vi "disk.vi"() -> ()   [LabVIEW 2016]
panel:
  out "free (bytes)":i64
  out "error out":errorcluster
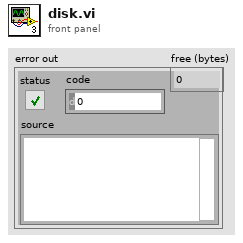
[diagram p1: front panel]
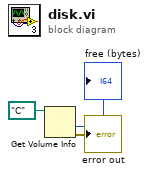
[diagram p0: block diagram]
diagram:
  n1 = Get Volume Info(11:path "C:/" ("path")) -> (0:→"error out":errorcluster, 1:→"free (bytes)":i64)  [unwired: 1 in, 4 out]
